vi "Help_URL.vi"() -> ()   [LabVIEW 2012]
panel:
  out "Help URL":string
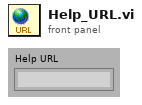
[diagram p1: front panel]
diagram:
